vi "NI PXI-4110 Programmable Power Supply Main Page.vi"(8 "error in (no error)":errorcluster, 11 "Node Ptr":T1 format="%.0x") -> (0 "error out":errorcluster)   [LabVIEW 2009, in "NI PXI-4110 Programmable Power Supply Custom Device.lvlib"]
uses:
  NI PXI-4110 Programmable Power Supply Custom Device.lvlib
  <vilib>/NI VeriStand/Custom Device API/Custom Device Item Ref.ctl
  <vilib>/NI VeriStand/Custom Device API/Get Item Property (String).vi
  4110_Global.vi
  <vilib>/NI VeriStand/Custom Device API/Set Item Property (String).vi
  <vilib>/NI VeriStand/Custom Device API/Custom Device API.lvlib
panel:
  in  "Name of Device in MAX":string
  in  "Add Current Chans":bool
  in  "Add Voltage Chans":bool
  in  "Header":cluster{"Section Name":string}={"Section Name"="PXI-4110  Settings"}
  in  "Description":string
  in  "Custom Device Name":string
  in  "Delete":bool
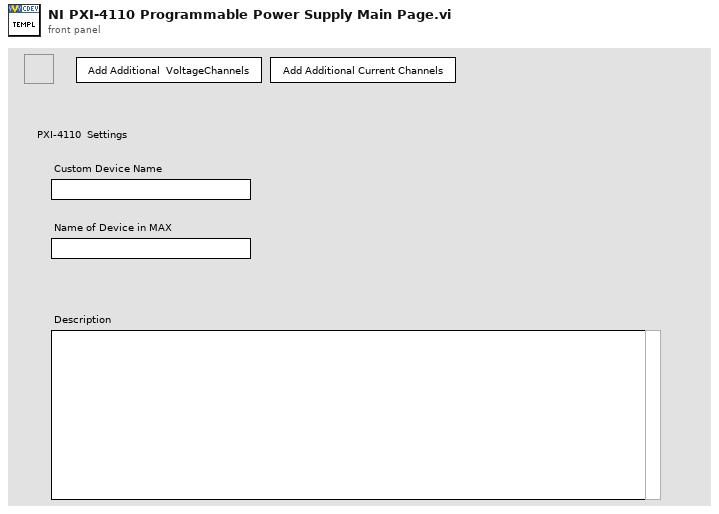
[diagram p1: front panel]
types:
  T1 = typedef "Custom Device API.lvlib/Custom Device Item Ref.ctl" = u64
  T2 = typedef "Custom Device API.lvlib/Custom Device Item Info.ctl" = cluster{"Name":string, "Is Channel":bool, "GUID":string}
  T3 = typedef "Custom Device API.lvlib/Custom Device Commands.ctl" = enum16{"Default", "Item renamed", "Shutdown"}
  T4 = typedef "niDCPower Sense.ctl" = i32
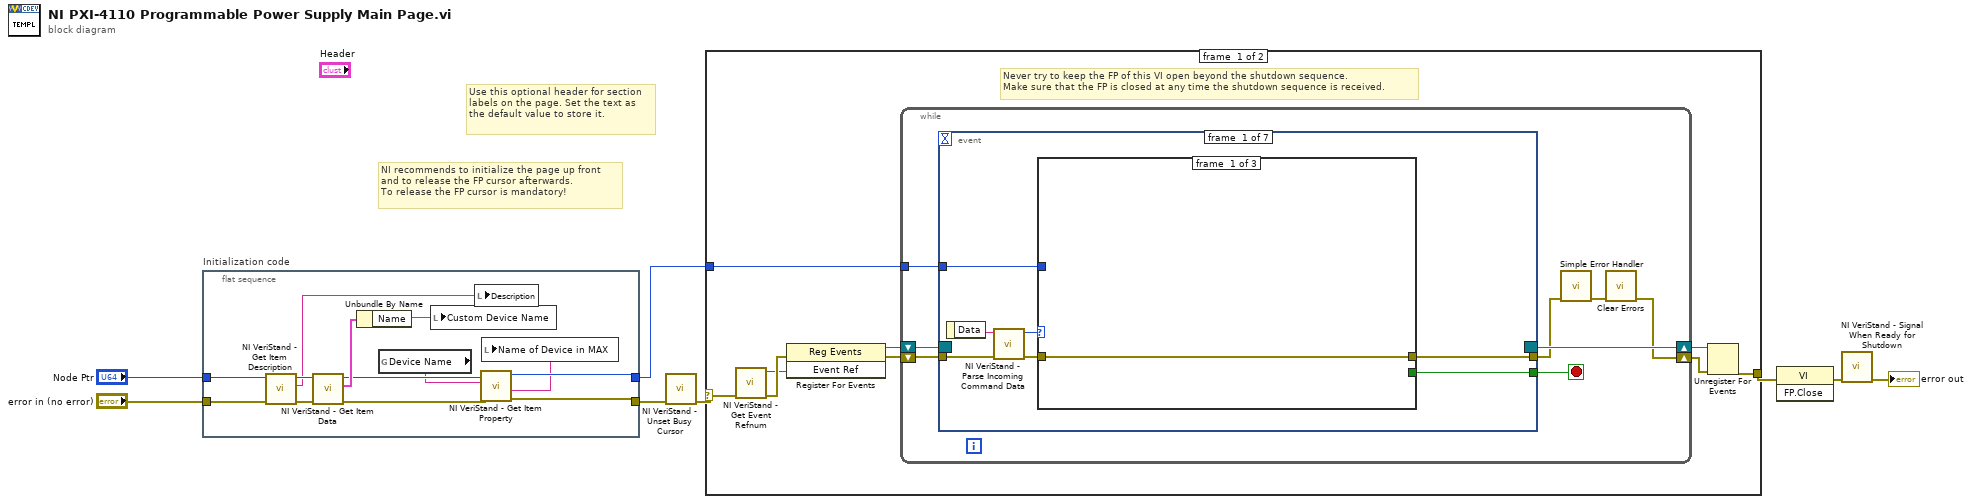
[diagram p0: block diagram]
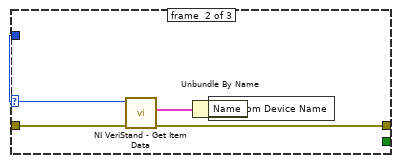
[diagram p2: hidden frame]
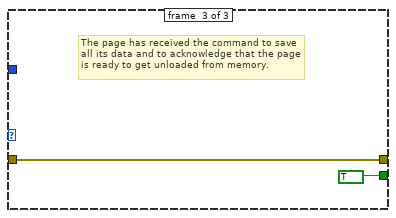
[diagram p3: hidden frame]
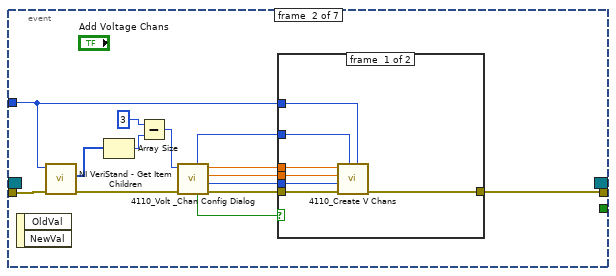
[diagram p4: hidden frame]
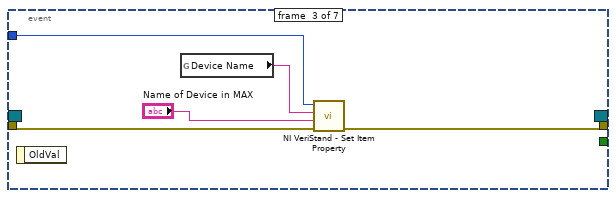
[diagram p6: hidden frame]
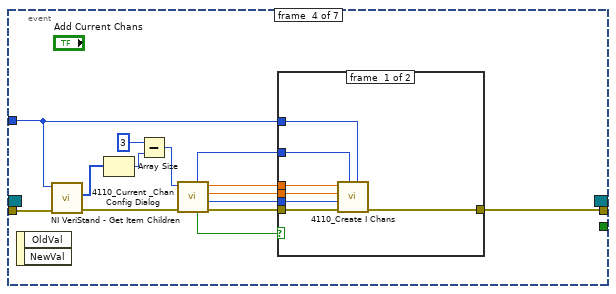
[diagram p7: hidden frame]
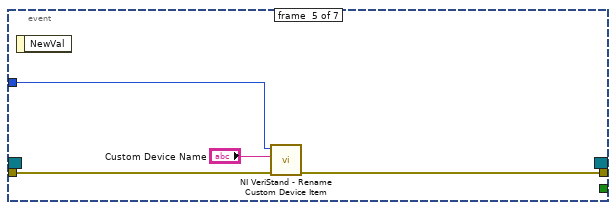
[diagram p9: hidden frame]
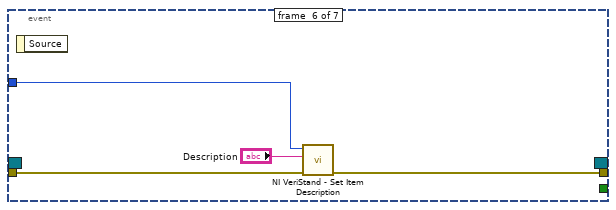
[diagram p10: hidden frame]
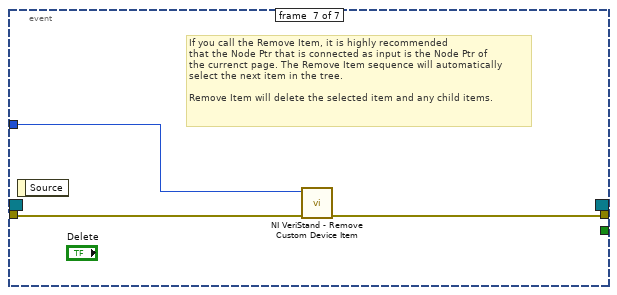
[diagram p11: hidden frame]
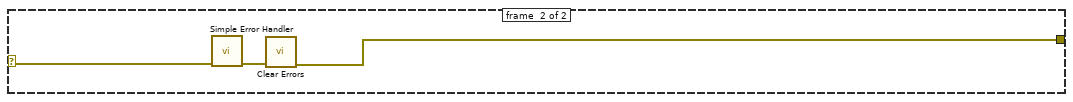
[diagram p12: hidden frame]
diagram:
  # "Use this optional header for section labels on the page. Set the text as the default value to store it."
  # "NI recommends to initialize the page up front\nand to release the FP cursor afterwards.\nTo release the FP cursor is mandatory!"
  n1 = flat-sequence "Initialization code" {
    tunnel: "error in (no error)" -> [w15]
    tunnel: "Node Ptr" -> [w16]
    tunnel: [w11] -> w4
    tunnel: [w12] -> w1
    frame #0 {
      n2 = call <vilib>:"NI VeriStand - Get Item Description.vi"("error in (no error)"=w15, "Item Ref in"=w16) -> ("error out"=w19:errorcluster, "Description"=w20:string, "Item Ref out"=w21:T1)  [unwired: 7 out]
      n3 = call <vilib>:"NI VeriStand - Get Item Data.vi"("error in (no error)"=w19, "Item Ref in"=w21) -> ("error out"=w14:errorcluster, "Item Info"=w18:T2, "Item Ref out"=w13:T1)  [unwired: 7 out]
      n4 = Unbundle By Name(w18) -> ("Name"=w17:string)
      n5 = global read "4110_Global.vi" "Device Name"() -> (w10:string)
      n6 = local write "Custom Device Name"(w17) -> ()
      n7 = local write "Description"(w20) -> ()
      n8 = call-poly <vilib>:"NI VeriStand - Get Item Property.vi"("error in (no error)"=w14, "Property Name"=w10, "Item Ref in"=w13) -> ("error out"=w11:errorcluster, "Value"=w9:string, "Item Ref out"=w12:T1)  [unwired: 5 in, 1 out]
      n9 = local write "Name of Device in MAX"(w9) -> ()
    }
  }
  n10 = call <vilib>:"NI VeriStand - Unset Busy Cursor.vi"("error in (no error)"=w4) -> ("error out"=w3:errorcluster)  [unwired: 10 out]
  n11 = case shown="No Error" w3 {
    selector: w3 -> [w22 w116]
    tunnel: [w27 w114] -> w8
    tunnel: w1 -> [w23 _]
    frame #0 {
      # "Never try to keep the FP of this VI open beyond the shutdown sequence.\nMake sure that the FP is closed at any time the shutdown sequence is received."
      n12 = call <vilib>:"NI VeriStand - Get Event Refnum.vi"("error in (no error)"=w22) -> ("error out"=w30:errorcluster, "Event Ref"=w26:refnum<user-event>)  [unwired: 9 out]
      n13 = register-events(error in=w30, w26) -> (reference out=w24:refnum<event-registration>, error out=w25:errorcluster)  [unwired: 1 in]
      n14 = while {
        tunnel: w23 -> [w34]
        shift-right: [w31] -> w28
        shift-left: w25 -> [w37]
        shift-right: [w38] -> w29
        shift-left: w24 -> [w36]
        stop <- w35 stop-if-true
        n15 = event shown="[3] \"Add Current Chans\": Value Change" {
          selector: w36 -> [_ _ _ _ _ _ _]
          dyn-events: [_ _ _ _ _ _ _] -> w38
          timeout: _ -> [_ _ _ _ _ _ _]
          tunnel: w37 -> [w45 w67 w80 w94 w106 w109 w113]
          tunnel: [w41 _ _ _ _ _ _] -> w35
          tunnel: [w40 w55 w76 w82 w105 w108 w112] -> w33
          tunnel: w34 -> [w39 w61 w79 w88 w104 w110 w111]
          event #0 {
            n16 = event-data() -> ("Data"=w44:string)  [unwired: 1 out]
            n17 = call <vilib>:"NI VeriStand - Parse Incoming Command Data.vi"("error in (no error)"=w45, "Data"=w44) -> ("error out"=w43:errorcluster, "Action"=w42:T3)  [unwired: 8 out]
            n18 = case shown="\"Shutdown\"" w42 {
              tunnel: w43 -> [w46 w51 w52]
              tunnel: [_ _ TRUE] -> w41
              tunnel: [w46 w48 w52] -> w40
              tunnel: w39 -> [_ w50 _]
              frame #0 {
              }
              frame #1 {
                n19 = call <vilib>:"NI VeriStand - Get Item Data.vi"("error in (no error)"=w51, "Item Ref in"=w50) -> ("error out"=w48:errorcluster, "Item Info"=w49:T2)  [unwired: 8 out]
                n20 = Unbundle By Name(w49) -> ("Name"=w47:string)
                n21 = local write "Custom Device Name"(w47) -> ()
              }
              frame #2 {
                # "The page has received the command to save all its data and to acknowledge that the page is ready to get unloaded from memory."
              }
            }
          }
          event #1 {
            n22 = event-data() -> ()  [unwired: 3 out]
            n23 = call <vilib>:"NI VeriStand - Get Item Children.vi"("error in (no error)"=w67, "Item Ref in"=w61) -> ("error out"=w66:errorcluster, "Child Refs"=w54:T1[])  [unwired: 6 in, 2 out]
            n24 = Array Size(array=w54) -> (size(s)=w64:i32)
            n25 = Subtract(x=3, y=w64) -> (x-y=w63:i32)
            n26 = call "4110_Volt _Chan Config Dialog.vi"("error in (no error)"=w66, "Data Entry Limits:Maximum"=w63) -> ("error out"=w56:errorcluster, "sense (out)"=w57:T4, "Current Limit (out)"=w58:dbl, "Initial Voltage Value (out)"=w59:dbl, "Cancel (out)"=w62:bool, "Number of Voltage Output Channels to Add? (out)"=w60:i16)  [unwired: 4 in]
            n27 = case shown="False" w62 {
              tunnel: w61 -> [w74 _]
              tunnel: w60 -> [w73 _]
              tunnel: w59 -> [w72 _]
              tunnel: w58 -> [w71 _]
              tunnel: w57 -> [w70 _]
              tunnel: w56 -> [w69 w75]
              tunnel: [w68 w75] -> w55
              frame #0 {
                n28 = call "4110_Create V Chans.vi"("Device Ref in"=w74, "# of V Channels to Add?"=w73, "error in"=w69, "sense"=w70, "Current Limit"=w71, "Init Value"=w72) -> ("error out"=w68:errorcluster)  [unwired: 5 in]
              }
              frame #1 {
                # "Canceled"
              }
            }
          }
          event #2 {
            n29 = event-data() -> ()  [unwired: 2 out]
            n30 = global read "4110_Global.vi" "Device Name"() -> (w78:string)
            n31 = call-poly <vilib>:"NI VeriStand - Set Item Property.vi"("error in (no error)"=w80, "Value"="Name of Device in MAX", "Property Name"=w78, "Item Ref in"=w79) -> ("error out"=w76:errorcluster)  [unwired: 5 in, 2 out]
          }
          event #3 {
            n32 = event-data() -> ()  [unwired: 3 out]
            n33 = call <vilib>:"NI VeriStand - Get Item Children.vi"("error in (no error)"=w94, "Item Ref in"=w88) -> ("error out"=w93:errorcluster, "Child Refs"=w81:T1[])  [unwired: 6 in, 2 out]
            n34 = Array Size(array=w81) -> (size(s)=w91:i32)
            n35 = Subtract(x=3, y=w91) -> (x-y=w90:i32)
            n36 = call "4110_Current _Chan Config Dialog.vi"("error in (no error)"=w93, "Data Entry Limits:Maximum"=w90) -> ("error out"=w83:errorcluster, "sense (out)"=w84:T4, "Voltage Limit (out)"=w85:dbl, "Initial Current Value (out)"=w86:dbl, "Cancel (out)"=w89:bool, "Number of Current Channels to Add? (out)"=w87:i16)  [unwired: 4 in]
            n37 = case shown="False" w89 {
              tunnel: w88 -> [w101 _]
              tunnel: w87 -> [w100 _]
              tunnel: w86 -> [w99 _]
              tunnel: w85 -> [w98 _]
              tunnel: w84 -> [w97 _]
              tunnel: w83 -> [w96 w102]
              tunnel: [w95 w102] -> w82
              frame #0 {
                n38 = call "4110_Create I Chans.vi"("Device Ref in"=w101, "# of I Channels to Add?"=w100, "error in"=w96, "sense"=w97, "Voltage Limit"=w98, "Init Value"=w99) -> ("error out"=w95:errorcluster)  [unwired: 5 in]
              }
              frame #1 {
                # "Canceled"
              }
            }
          }
          event #4 {
            n39 = event-data() -> ()  [unwired: 2 out]
            n40 = call <vilib>:"NI VeriStand - Rename Custom Device Item.vi"("error in (no error)"=w106, "New Name"="Custom Device Name", "Item Ref in"=w104) -> ("error out"=w105:errorcluster)  [unwired: 8 out]
          }
          event #5 {
            n41 = event-data() -> ()  [unwired: 2 out]
            n42 = call <vilib>:"NI VeriStand - Set Item Description.vi"("error in (no error)"=w109, "Description"="Description", "Item Ref in"=w110) -> ("error out"=w108:errorcluster)  [unwired: 8 out]
          }
          event #6 {
            # "If you call the Remove Item, it is highly recommended\nthat the Node Ptr that is connected as input is the Node Ptr of\nthe currenct page. The Remove Item sequence will automatically\nselect the next item in the tree.\n\nRemove Item will delete the selected item and any child items."
            n43 = event-data() -> ()  [unwired: 2 out]
            n44 = call <vilib>:"NI VeriStand - Remove Custom Device Item.vi"("error in (no error)"=w113, "Item Ref in"=w111) -> ("error out"=w112:errorcluster)  [unwired: 1 in, 8 out]
          }
        }
        n45 = call <vilib>:"Simple Error Handler.vi"("error in (no error)"=w33) -> ("error out"=w32:errorcluster)  [unwired: 1 in, 7 out]
        n46 = call <vilib>:"Clear Errors.vi"("error in (no error)"=w32) -> ("error out"=w31:errorcluster)  [unwired: 6 out]
      }
      n47 = Unregister For Events(event registration refnum=w29, error in=w28) -> (error out=w27:errorcluster)
    }
    frame #1 {
      n48 = call <vilib>:"Simple Error Handler.vi"("error in (no error)"=w116) -> ("error out"=w115:errorcluster)  [unwired: 1 in, 7 out]
      n49 = call <vilib>:"Clear Errors.vi"("error in (no error)"=w115) -> ("error out"=w114:errorcluster)  [unwired: 6 out]
    }
  }
  n50 = invoke class="VI" method="FP.Close"(error in=w8) -> (error out=w7:errorcluster)  [unwired: 2 in, 2 out]
  n51 = call <vilib>:"NI VeriStand - Signal When Ready for Shutdown.vi"("error in (no error)"=w7) -> ("error out"=→"error out":errorcluster)  [unwired: 10 out]
